vi "_Save RT Table.vi"(4 "error in (no error)":errorcluster, 6 "Table":dbl[][](array[numeric]), 7 "key":string) -> (0 "error out":errorcluster)   [LabVIEW 2012]
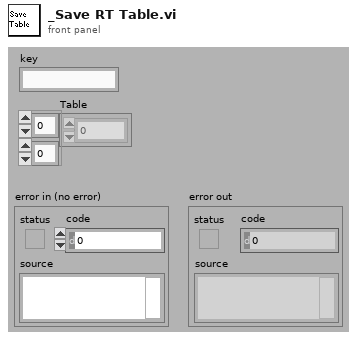
[diagram p1: front panel]
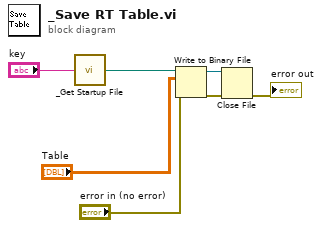
[diagram p0: block diagram]
diagram:
  n1 = call "_Get Startup File.vi"("FileName"="key") -> ("FilePath"=w2:path)
  n2 = Write to Binary File(file (use dialog)=w2, data="Table", error in="error in (no error)") -> (refnum out=w5:refnum<file>, error out=w6:errorcluster)  [unwired: 4 out]
  n3 = Close File(refnum=w5, error in=w6) -> (error out=→"error out":errorcluster)  [unwired: 1 out]
